vi "Get PTR With Limits.vi"(8 "error in":errorcluster, 11 "Path to STDF file":path) -> (0 "error out":errorcluster, 2 "Part_CNT":u32, 3 "PTRs W/Limits":refnum<class "PTR.lvclass">[](array[class]))   [LabVIEW 2018, in "STDF File Parser.lvclass"]
uses:
  STDF File Parser.lvclass
  <userlib>/STDF/PTR/PTR.lvclass
  <userlib>/STDF/Common/Typedefs/Record type.ctl
  <userlib>/STDF/PCR/Cast Record to PCR.vi
  <vilib>/Utility/error.llb/Error Cluster From Error Code.vi
  <userlib>/STDF/PTR/Cast Record to PTR.vi
  <vilib>/ErrorRing/Error Ring.xnode
  <userlib>/STDF/STDF Reader/STDF Reader.lvclass
  <userlib>/STDF/PCR/PCR.lvclass
  <userlib>/STDF/STDF.lvlib
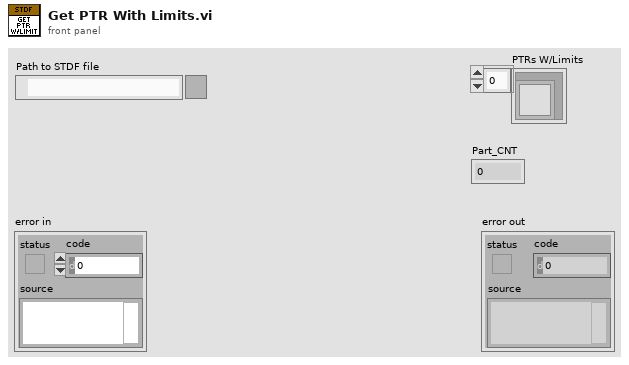
[diagram p1: front panel]
types:
  T1 = typedef "STDF.lvlib/Record type.ctl" = enum16{"INVALID", "ATR", "BPS", "DTR", "EPS", "FAR", "FTR", "GDR", "HBR", "MIR", "MPR", "MRR", "PCR", "PGR", "PIR", "PLR", "PMR", "PRR", "PTR", "RDR", "SBR", "SDR", "TSR", "WCR", "WIR", "WRR"}
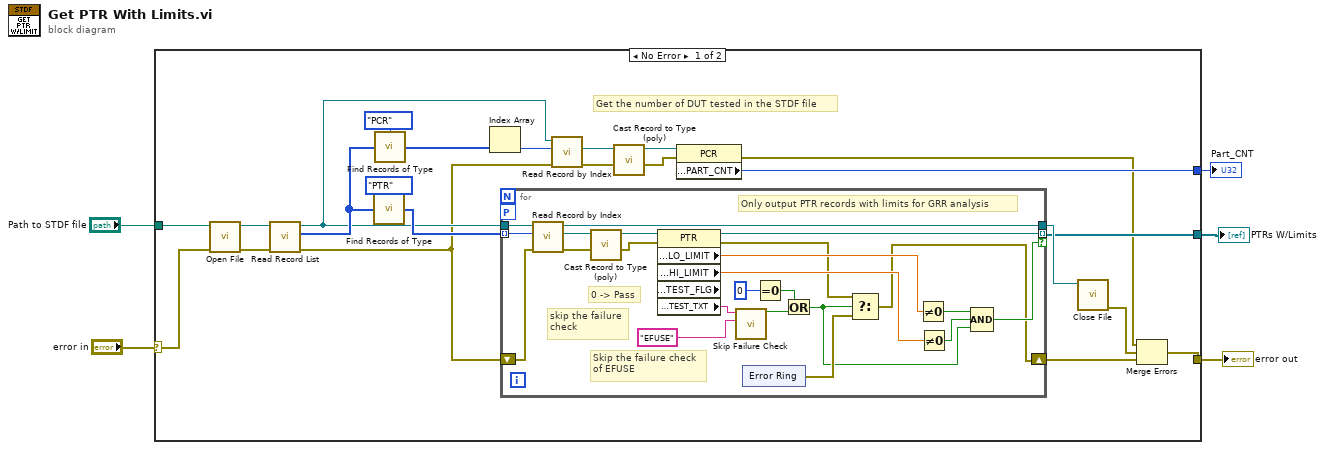
[diagram p0: block diagram]
diagram:
  n1 = case shown="No Error" "error in" {
    selector: "error in" -> [w21 w57]
    tunnel: "Path to STDF file" -> [w26 _]
    tunnel: [w22 _] -> w4
    tunnel: [w18 w57] -> w3
    tunnel: [w7 _] -> w1
    frame No Error {
      # "Get the number of DUT tested in the STDF file"
      n2 = call <userlib>:"Open File.vi"("error in (no error)"=w21, "File path"=w26) -> ("error out"=w27:errorcluster, "STDF Reader"=w28:refnum<class "STDF Reader.lvclass">)  [unwired: 8 in]
      n3 = call-dynamic "Read Record List.vi"("error in (no error)"=w27, "STDF Reader in"=w28) -> ("error out"=w12:errorcluster, "Record list"=w17:T1[], "STDF Reader out"=w14:refnum<class "STDF Reader.lvclass">)  [unwired: 7 in]
      n4 = call <userlib>:"Find Records of Type.vi"("Record list"=w17, "Record type"=Record_type."PTR") -> ("Record indices"=w24:i32[])
      n5 = call <userlib>:"Find Records of Type.vi"("Record list"=w17, "Record type"=Record_type."PCR") -> ("Record indices"=w15:i32[])
      n6 = Index Array(array=w15) -> (element=w13:i32)  [unwired: 1 in]
      n7 = for "Get records and cast to specific type" {
        shift-right: [w31] -> w19
        shift-left: w12 -> [w50]
        tunnel: w24 -> [w48] mode=indexing
        tunnel: [w43] -> w22 mode=indexing if=w36
        workers-P: _ -> [_]
        tunnel: w14 -> [w51]
        tunnel: [w49] -> w23
        # "Only output PTR records with limits for GRR analysis"
        # "skip the failure\ncheck"
        # "Skip the failure check\nof EFUSE"
        # "0 -> Pass"
        n8 = call-dynamic "Read Record by Index.vi"("error in (no error)"=w50, "Index"=w48, "STDF Reader in"=w51) -> ("error out"=w47:errorcluster, "Record"=w46:refnum<class "Record.lvclass">, "STDF Reader out"=w49:refnum<class "STDF Reader.lvclass">)  [unwired: 6 in]
        n9 = call-poly <userlib>:"Cast Record to Type (poly).vi"("error in (no error)"=w47, "Record in"=w46) -> ("error out"=w44:errorcluster, "PTR out"=w45:refnum<class "PTR.lvclass">)  [unwired: 8 in]
        n10 = property class="PTR" props=["Accessors:LO_LIMIT", "Accessors:HI_LIMIT", "Accessors:TEST_FLG", "Accessors:TEST_TXT"](reference=w45, error in=w44) -> (reference out=w43:refnum<class "PTR.lvclass">, error out=w40:errorcluster, "Accessors:LO_LIMIT"=w42:sgl, "Accessors:HI_LIMIT"=w41:sgl, "Accessors:TEST_TXT"=w29:string)  [unwired: 1 out]
        n11 = call "Skip Failure Check.vi"("Test Name Prefix"="EFUSE", "Test Name Input"=w29) -> ("Skip Failure Check?"=w33:bool)  [unwired: 9 in]
        n12 = xnode "Error Ring"() -> ("error out"=w39:errorcluster)
        n13 = Equal To 0?(x=0) -> (x = 0?=w34:bool)
        n14 = Or(x=w34, y=w33) -> (x .or. y?=w32:bool)
        n15 = Select(t=w40, s=w32, f=w39) -> (s? t:f=w31:errorcluster)
        n16 = Not Equal To 0?(x=w42) -> (x != 0?=w38:bool)
        n17 = Not Equal To 0?(x=w41) -> (x != 0?=w37:bool)
        n18 = Compound Arithmetic op=AND(w38, w37, w32) -> (w36:bool)
      }
      n19 = call-dynamic "Read Record by Index.vi"("error in (no error)"=w12, "Index"=w13, "STDF Reader in"=w14) -> ("error out"=w11:errorcluster, "Record"=w10:refnum<class "Record.lvclass">)  [unwired: 6 in, 1 out]
      n20 = call-poly <userlib>:"Cast Record to Type (poly).vi"("error in (no error)"=w11, "Record in"=w10) -> ("error out"=w8:errorcluster, "PCR out"=w9:refnum<class "PCR.lvclass">)  [unwired: 8 in]
      n21 = property class="PCR"(reference=w9, error in=w8) -> (error out=w6:errorcluster, "Accessors:PART_CNT"=w7:u32)  [unwired: 1 out]
      n22 = call-dynamic "Close File.vi"("STDF Reader in"=w23) -> ("error out"=w20:errorcluster)  [unwired: 8 in, 2 out]
      n23 = Merge Errors(w6, w20, w19) -> (w18:errorcluster)
    }
    frame Error {
    }
  }
  "PTRs W/Limits" <- w4
  "error out" <- w3
  "Part_CNT" <- w1
